vi "Steve's Autoomononiss.vi"(8 "error in (no error)":errorcluster) -> (0 "error out":errorcluster)   [LabVIEW 2014]
uses:
  <vilib>/Rock Robotics/WPI/RobotDrive/WPI_RobotDriveGetSetRefNum.vi
  <vilib>/Rock Robotics/WPI/RobotDrive/WPI_RobotDriveMecanumDrive_Cartesian.vi
  <vilib>/Rock Robotics/Network Tables/SD Write Numeric Array.vi
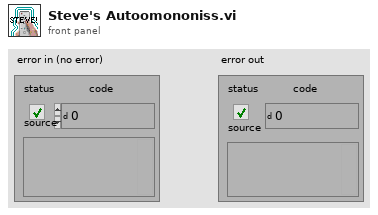
[diagram p1: front panel]
types:
  T1 = typedef "WPI_RobotDriveDevRef.ctl" = cluster{"DevStatus":errorcluster, "Motors[]":T2[], "Square Inputs":bool, "Max Output":dbl}
  T2 = typedef "WPI_MotorControlDeviceRef.ctl" = cluster{"DeviceStatus":errorcluster, "Type":T3, "PWM":cluster{"Controller":T4, "PWM Channel":T5, "DeadBand":T6}, "CAN":cluster{"Device Number":u8, "Control Mode":T7, "Semaphore":T8, "Max Vout":dbl, "TalonSRX Control Mode":T9}, "Invert":bool, "TransformRef":T10, "InvTransformRef":T10}
  T3 = typedef "WPI_MotorControlType.ctl" = enum16{"PWM", "CAN", "CANTalonSRX"}
  T4 = typedef "FPGA_TypedefDigitalModule.ctl" = enum16{"Controller 1"}
  T5 = typedef "FPGA_DIOPWMChannel.ctl" = enum8{"PWM 0", "PWM 1", "PWM 2", "PWM 3", "PWM 4", "PWM 5", "PWM 6", "PWM 7", "PWM 8", "PWM 9", "PWM MXP 0", "PWM MXP 1", "PWM MXP 2", "PWM MXP 3", "PWM MXP 4", "PWM MXP 5", "PWM MXP 6", "PWM MXP 7", "PWM MXP 8", "PWM MXP 9", "Invalid"}
  T6 = typedef "WPI_PWMDeadband.ctl" = cluster{"Name":string, "maxPositivePwm":i32, "minPositivePwm":i32, "centerPwm":i32, "maxNegativePwm":i32, "minNegativePwm":i32, "angularRange":u16}
  T7 = typedef "WPI_CANJaguar_ControlMode.ctl" = enum8{"Percent VBus", "Current", "Speed", "Position", "Voltage"}
  T8 = typedef "Semaphore RefNum" = refnum<k1>
  T9 = typedef "WPI_CANTalonSRX_APIControlMode.ctl" = enum8{"Percent VBus", "Speed", "Position", "Slave", "Unchanged / Invalid"}
  T10 = typedef "WPI_PWMTransform_ConPane.ctl" = refnum<vi>
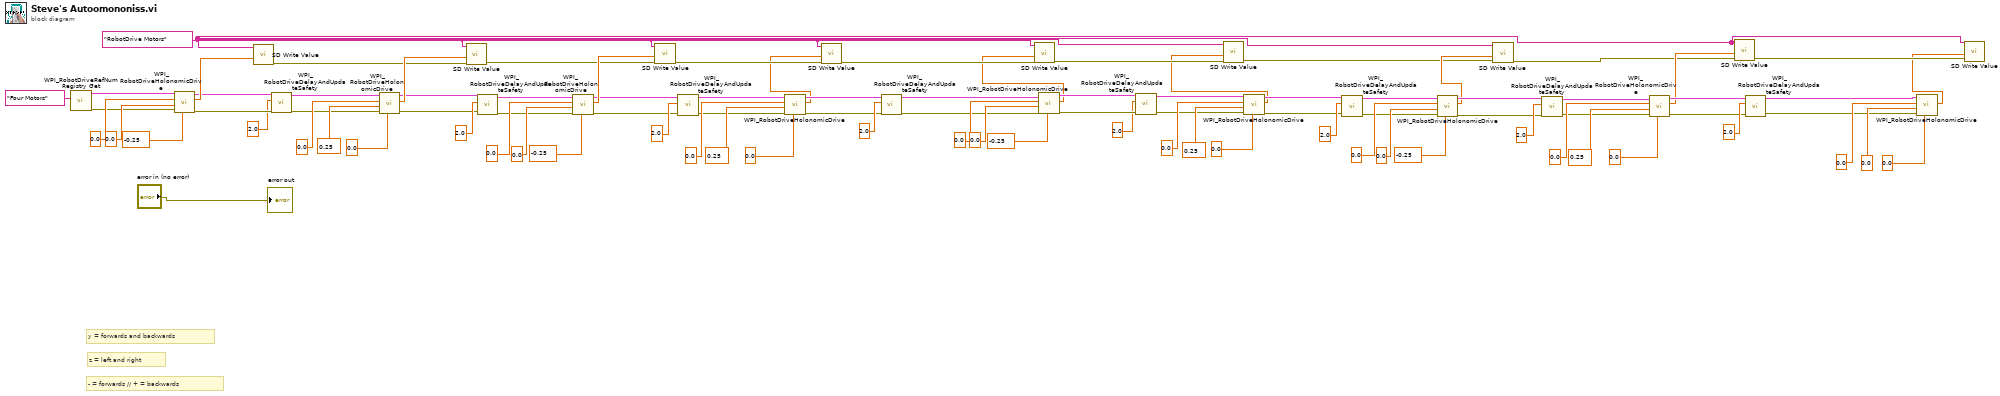
[diagram p0: block diagram]
diagram:
  w12 = "RobotDrive Motors" ("Name")
  # "- = forwards // + = backwards"
  # "z = left and right"
  # "y = forwards and backwards"
  n1 = call <vilib>:"WPI_RobotDriveRefNum Registry Get.vi"("refnum name"="Four Motors") -> ("error out"=w81:errorcluster, "RobotDriveDevRef"=w88:T1)  [unwired: 1 in, 8 out]
  n2 = call-poly <vilib>:"WPI_RobotDriveHolonomicDrive.vi"("Rotation"=-0.25 ("X"), "error in (no error)"=w81, "Y"=0.0 ("X"), "X"=0.0, "RobotDriveDevRef"=w88) -> ("error out"=w75:errorcluster, "Motor Values"=w84:dbl[], "RobotDriveDevRef"=w77:T1)  [unwired: 4 in]
  n3 = call-poly <vilib>:"SD Write Value.vi"("Numeric Array"=w84, "Name"=w12) -> ("error out"=w82:errorcluster)  [unwired: 8 in, 1 out]
  n4 = call <vilib>:"WPI_RobotDriveDelayAndUpdateSafety.vi"("error in (no error)"=w75, "Delay (s)"=2.0, "RobotDriveDevRef"=w77) -> ("error out"=w74:errorcluster, "RobotDriveDevRef 2"=w76:T1)  [unwired: 7 in]
  n5 = call-poly <vilib>:"WPI_RobotDriveHolonomicDrive.vi"("Rotation"=0.0 ("X"), "error in (no error)"=w74, "Y"=0.25 ("X"), "X"=0.0, "RobotDriveDevRef"=w76) -> ("error out"=w64:errorcluster, "Motor Values"=w83:dbl[], "RobotDriveDevRef"=w72:T1)  [unwired: 4 in]
  n6 = call-poly <vilib>:"SD Write Value.vi"("error in"=w82, "Numeric Array"=w83, "Name"=w12) -> ("error out"=w65:errorcluster)  [unwired: 7 in, 1 out]
  n7 = call <vilib>:"WPI_RobotDriveDelayAndUpdateSafety.vi"("error in (no error)"=w64, "Delay (s)"=2.0, "RobotDriveDevRef"=w72) -> ("error out"=w63:errorcluster, "RobotDriveDevRef 2"=w71:T1)  [unwired: 7 in]
  n8 = call-poly <vilib>:"WPI_RobotDriveHolonomicDrive.vi"("Rotation"=-0.25 ("X"), "error in (no error)"=w63, "Y"=0.0 ("X"), "X"=0.0, "RobotDriveDevRef"=w71) -> ("error out"=w29:errorcluster, "Motor Values"=w70:dbl[], "RobotDriveDevRef"=w62:T1)  [unwired: 4 in]
  n9 = call-poly <vilib>:"SD Write Value.vi"("error in"=w65, "Numeric Array"=w70, "Name"=w12) -> ("error out"=w20:errorcluster)  [unwired: 7 in, 1 out]
  n10 = call <vilib>:"WPI_RobotDriveDelayAndUpdateSafety.vi"("error in (no error)"=w29, "Delay (s)"=2.0, "RobotDriveDevRef"=w62) -> ("error out"=w28:errorcluster, "RobotDriveDevRef 2"=w60:T1)  [unwired: 7 in]
  n11 = call-poly <vilib>:"WPI_RobotDriveHolonomicDrive.vi"("Rotation"=0.0 ("X"), "error in (no error)"=w28, "Y"=0.25 ("X"), "X"=0.0, "RobotDriveDevRef"=w60) -> ("error out"=w27:errorcluster, "Motor Values"=w19:dbl[], "RobotDriveDevRef"=w56:T1)  [unwired: 4 in]
  n12 = call-poly <vilib>:"SD Write Value.vi"("error in"=w20, "Numeric Array"=w19, "Name"=w12) -> ("error out"=w22:errorcluster)  [unwired: 7 in, 1 out]
  n13 = call <vilib>:"WPI_RobotDriveDelayAndUpdateSafety.vi"("error in (no error)"=w27, "Delay (s)"=2.0, "RobotDriveDevRef"=w56) -> ("error out"=w26:errorcluster, "RobotDriveDevRef 2"=w30:T1)  [unwired: 7 in]
  n14 = call-poly <vilib>:"WPI_RobotDriveHolonomicDrive.vi"("Rotation"=-0.25 ("X"), "error in (no error)"=w26, "Y"=0.0 ("X"), "X"=0.0, "RobotDriveDevRef"=w30) -> ("error out"=w46:errorcluster, "Motor Values"=w18:dbl[], "RobotDriveDevRef"=w48:T1)  [unwired: 4 in]
  n15 = call-poly <vilib>:"SD Write Value.vi"("error in"=w22, "Numeric Array"=w18, "Name"=w12) -> ("error out"=w21:errorcluster)  [unwired: 7 in, 1 out]
  n16 = call <vilib>:"WPI_RobotDriveDelayAndUpdateSafety.vi"("error in (no error)"=w46, "Delay (s)"=2.0, "RobotDriveDevRef"=w48) -> ("error out"=w45:errorcluster, "RobotDriveDevRef 2"=w47:T1)  [unwired: 7 in]
  n17 = call-poly <vilib>:"WPI_RobotDriveHolonomicDrive.vi"("Rotation"=0.0 ("X"), "error in (no error)"=w45, "Y"=0.25 ("X"), "X"=0.0, "RobotDriveDevRef"=w47) -> ("error out"=w37:errorcluster, "Motor Values"=w17:dbl[], "RobotDriveDevRef"=w43:T1)  [unwired: 4 in]
  n18 = call-poly <vilib>:"SD Write Value.vi"("error in"=w21, "Numeric Array"=w17, "Name"=w12) -> ("error out"=w15:errorcluster)  [unwired: 7 in, 1 out]
  n19 = call <vilib>:"WPI_RobotDriveDelayAndUpdateSafety.vi"("error in (no error)"=w37, "Delay (s)"=2.0, "RobotDriveDevRef"=w43) -> ("error out"=w36:errorcluster, "RobotDriveDevRef 2"=w42:T1)  [unwired: 7 in]
  n20 = call-poly <vilib>:"WPI_RobotDriveHolonomicDrive.vi"("Rotation"=-0.25 ("X"), "error in (no error)"=w36, "Y"=0.0 ("X"), "X"=0.0, "RobotDriveDevRef"=w42) -> ("error out"=w3:errorcluster, "Motor Values"=w16:dbl[], "RobotDriveDevRef"=w35:T1)  [unwired: 4 in]
  n21 = call-poly <vilib>:"SD Write Value.vi"("error in"=w15, "Numeric Array"=w16, "Name"=w12) -> ("error out"=w13:errorcluster)  [unwired: 7 in, 1 out]
  n22 = call <vilib>:"WPI_RobotDriveDelayAndUpdateSafety.vi"("error in (no error)"=w3, "Delay (s)"=2.0, "RobotDriveDevRef"=w35) -> ("error out"=w4:errorcluster, "RobotDriveDevRef 2"=w33:T1)  [unwired: 7 in]
  n23 = call-poly <vilib>:"WPI_RobotDriveHolonomicDrive.vi"("Rotation"=0.0 ("X"), "error in (no error)"=w4, "Y"=0.25 ("X"), "X"=0.0, "RobotDriveDevRef"=w33) -> ("error out"=w5:errorcluster, "Motor Values"=w14:dbl[], "RobotDriveDevRef"=w32:T1)  [unwired: 4 in]
  n24 = call-poly <vilib>:"SD Write Value.vi"("error in"=w13, "Numeric Array"=w14, "Name"=w12) -> ("error out"=w7:errorcluster)  [unwired: 7 in, 1 out]
  n25 = call <vilib>:"WPI_RobotDriveDelayAndUpdateSafety.vi"("error in (no error)"=w5, "Delay (s)"=2.0, "RobotDriveDevRef"=w32) -> ("error out"=w6:errorcluster, "RobotDriveDevRef 2"=w11:T1)  [unwired: 7 in]
  n26 = call-poly <vilib>:"WPI_RobotDriveHolonomicDrive.vi"("Rotation"=0.0 ("X"), "error in (no error)"=w6, "Y"=0.0 ("X"), "X"=0.0, "RobotDriveDevRef"=w11) -> ("Motor Values"=w2:dbl[])  [unwired: 4 in, 2 out]
  n27 = call-poly <vilib>:"SD Write Value.vi"("error in"=w7, "Numeric Array"=w2, "Name"=w12) -> ()  [unwired: 7 in, 2 out]
  "error out" <- "error in (no error)"
